vi "Bitwise.vi"(8 "error in":errorcluster, 11 "Number in":u16 format="%x") -> (0 "error out":errorcluster, 2 "Array":i32[](array[numeric]), 3 "Numeric out":u16 format="%b")   [LabVIEW 2019]
panel:
  out "Boolean array":bool[](array[boolean])
  out "index of element":i32
  out "x .and. y?":bool[](array[boolean])
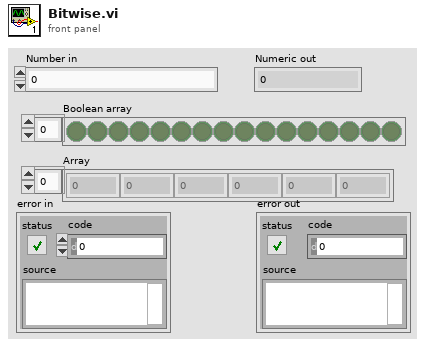
[diagram p1: front panel]
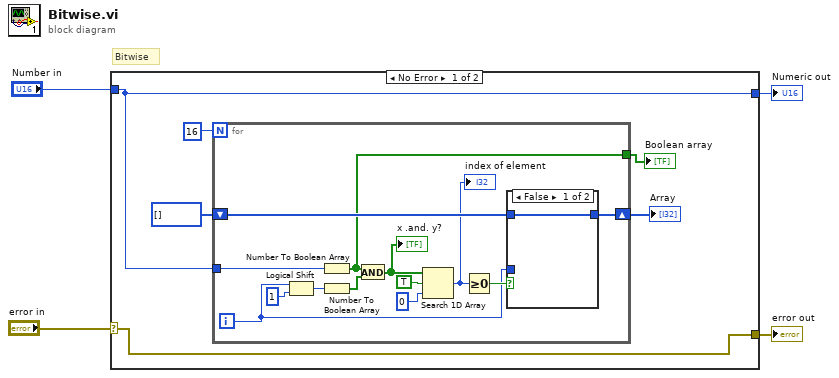
[diagram p0: block diagram]
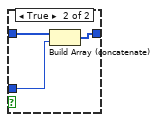
[diagram p2: hidden frame]
diagram:
  # "Bitwise"
  n1 = case shown="No Error" "error in" {
    selector: "error in" -> [w6 w29]
    tunnel: "Number in" -> [w5 w28]
    tunnel: [w6 w29] -> w3
    tunnel: [w5 w28] -> w1
    frame No Error {
      n2 = for {
        N: 16 -> [_]
        tunnel: w5 -> [w22]
        shift-right: [w13] -> w8
        shift-left: i32[] [] -> [w15]
        tunnel: [w12] -> w7
        i -> [w14]
        n3 = Logical Shift(y=w14, x=i16 1 ("y")) -> (x << y=w21:i16)
        n4 = Number To Boolean Array(number=w22) -> (Boolean array=w12:bool[])
        n5 = Number To Boolean Array(number=w21) -> (Boolean array=w20:bool[])
        n6 = And(x=w12, y=w20) -> (x .and. y?=w19:bool[])
        "x .and. y?" <- w19
        n7 = Search 1D Array(1D array=w19, element=TRUE, start index (0)=0) -> (index of element=w11:i32)
        "index of element" <- w11
        n8 = Greater Or Equal To 0?(x=w11) -> (x >= 0?=w16:bool)
        n9 = case shown="False" w16 {
          tunnel: w15 -> [w24 w27]
          tunnel: w14 -> [_ w26]
          tunnel: [w24 w25] -> w13
          frame False {
          }
          frame True {
            n10 = Build Array (concatenate)(w27, w26) -> (w25:i32[])
          }
        }
      }
      "Array" <- w8
      "Boolean array" <- w7
    }
    frame Error {
    }
  }
  "error out" <- w3
  "Numeric out" <- w1
